vi "is_paused.vi"(7 "url":string, 8 "error in (no error)":errorcluster, 11 "client handle":T1) -> (0 "error out":errorcluster, 2 "paused":bool, 3 "client handle out":T1)   [LabVIEW 2022 SP3]
uses:
  <vilib>/httpClient/ClientHandle.ctl
  <vilib>/httpClient/LabVIEWHTTPClient.lvlib
panel:
  out "concatenated string":string
  out "body":string
  out "value":cluster{"status":i32}
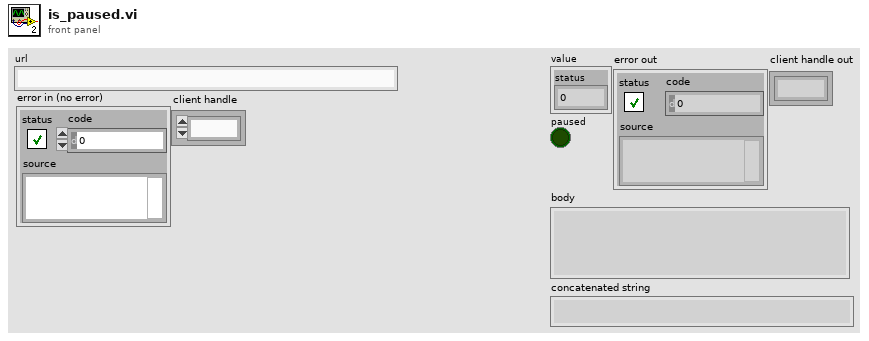
[diagram p1: front panel]
types:
  T1 = typedef "LabVIEWHTTPClient.lvlib/ClientHandle.ctl" = refnum<k1>
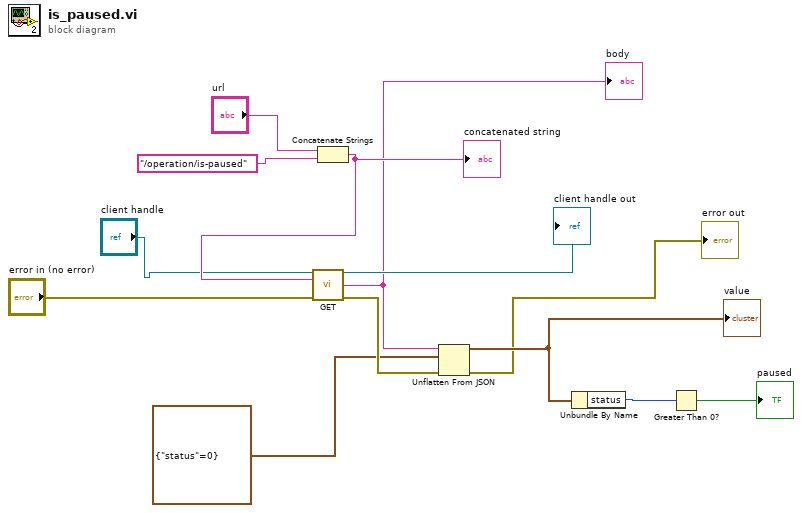
[diagram p0: block diagram]
diagram:
  n1 = Concatenate Strings("url", "/operation/is-paused" ("string")) -> (w11:string)
  "concatenated string" <- w11
  n2 = call <vilib>:"GET.vi"("client handle"="client handle", "url"=w11, "error in (no error)"="error in (no error)") -> ("client handle out"=→"client handle out":T1, "body"=w9:string, "error out"=w8:errorcluster)  [unwired: 9 in, 1 out]
  "body" <- w9
  n3 = Unflatten From JSON(JSON string=w9, type and defaults=cluster{"status":i32} {"status"=0}, error in (no error)=w8) -> (value=w6:cluster{"status":i32}, error out=→"error out":errorcluster)  [unwired: 4 in]
  "value" <- w6
  n4 = Unbundle By Name(w6) -> ("status"=w5:i32)
  n5 = Greater Than 0?(x=w5) -> (x > 0?=→"paused":bool)
